vi "Trivial_client.vi"() -> (0 "Difference":dbl format="%.2f", 1 "Server time":dbl format="%.2f")   [LabVIEW 2020]
doc: "This is an example of using features of the VI Server as a client. It shows how you might browse from one or more applications that may be exporting data from one or more data stations. \n\nThe example shows how to query a server for its list of exported VIs, how to get references to the VIs, and how call them with the Call By Reference function."
uses:
  Anemometry/Anemometry Sub Vis/Globals/Preference_global.vi
panel:
  out "Iterations":i32
  out "error Out":errorcluster
  in  "trivial.vi type":refnum<vi>
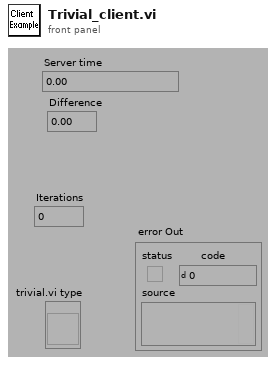
[diagram p1: front panel]
types:
  T1 = typedef "Server_Comms.ctl" = enum16{"Do Not Link To Server", "Server Link Healthy"}
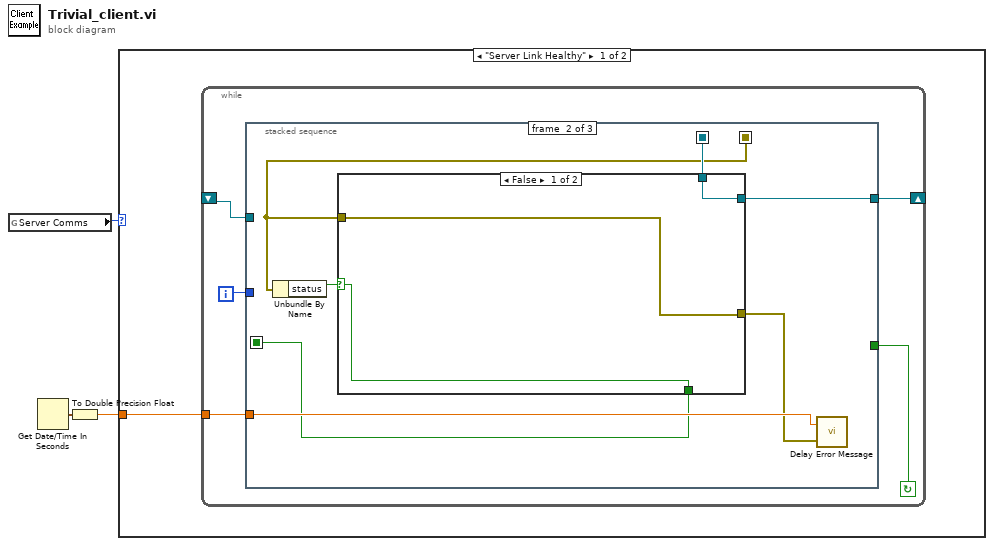
[diagram p0: block diagram]
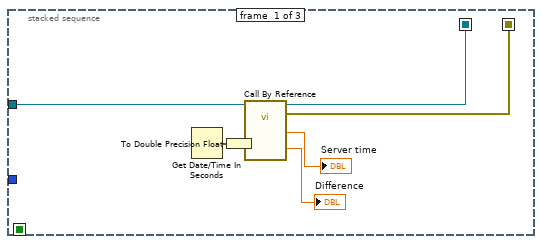
[diagram p2: hidden frame]
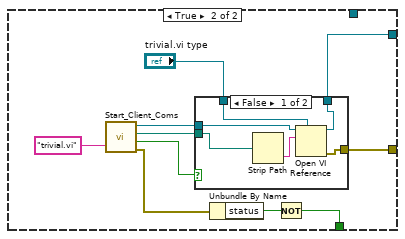
[diagram p3: hidden frame]
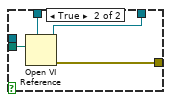
[diagram p4: hidden frame]
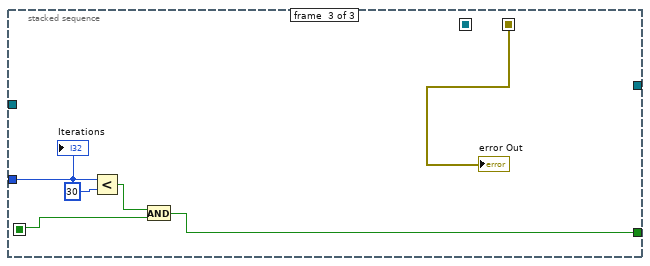
[diagram p5: hidden frame]
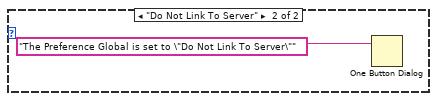
[diagram p6: hidden frame]
diagram:
  n1 = global read "Preference_global.vi" "Server Comms"() -> (w3:T1)
  n2 = Get Date/Time In Seconds() -> (seconds since 1Jan1904=w2:timestamp)
  n3 = To Double Precision Float(number=w2) -> (double precision float=w1:dbl)
  n4 = case shown="\"Server Link Healthy\"" w3 {
    tunnel: w1 -> [w4 _]
    frame "Server Link Healthy" {
      n5 = while {
        shift-left: _ -> [w9]
        shift-right: [w8] -> _
        tunnel: w4 -> [w5]
        i -> [w7]
        stop <- w6 continue-if-true
        n6 = stacked-sequence {
          seq-local: [w11 _ _] -> [_ w22 _]
          seq-local: [w13 _ _] -> [_ w20 w48]
          seq-local: [_ w17 _] -> [_ _ w49]
          tunnel: w9 -> [w12 _ _]
          tunnel: [_ w23 _] -> w8
          tunnel: w7 -> [_ _ w50]
          tunnel: [_ _ w47] -> w6
          tunnel: w5 -> [_ w19 _]
          frame #0 {
            n7 = Get Date/Time In Seconds() -> (seconds since 1Jan1904=w10:timestamp)
            n8 = To Double Precision Float(number=w10) -> (double precision float=w14:dbl)
            n9 = call-by-ref "?"(reference=w12, "Client time"=w14) -> (reference out=w11:refnum<vi>, error out=w13:errorcluster, "Server time"=→"Server time":dbl, "Difference"=→"Difference":dbl)  [unwired: 1 in]
          }
          frame #1 {
            n10 = Unbundle By Name(w20) -> ("status"=w21:bool)
            n11 = case shown="False" w21 {
              selector: w21 -> [w24 _]
              tunnel: [w26 w32] -> w23
              tunnel: w22 -> [w26 _]
              tunnel: [w25 w30] -> w18
              tunnel: w20 -> [w25 _]
              tunnel: [w24 w27] -> w17
              frame False {
              }
              frame True {
                n12 = call "Start_Client_Coms.vi"("VI name to run on server"="trivial.vi") -> ("LabVIEW application reference"=w34:refnum<vi>, "Checked VI name"=w31:path, "Local Call"=w33:bool, "Error cluster"=w28:errorcluster)  [unwired: 1 in]
                n13 = case shown="False" w33 {
                  tunnel: [w39 w46] -> w32
                  tunnel: "trivial.vi type" -> [w38 w45]
                  tunnel: w31 -> [w40 w44]
                  tunnel: w34 -> [w37 _]
                  tunnel: [w41 w43] -> w30
                  frame False {
                    n14 = Strip Path(path=w40) -> (name=w42:string)  [unwired: 1 out]
                    n15 = Open VI Reference(type specifier VI Refnum (for type only)=w38, application reference (local)=w37, vi path=w42) -> (vi reference=w39:refnum<vi>, error out=w41:errorcluster)  [unwired: 1 in, 2 out]
                  }
                  frame True {
                    n16 = Open VI Reference(type specifier VI Refnum (for type only)=w45, vi path=w44) -> (vi reference=w46:refnum<vi>, error out=w43:errorcluster)  [unwired: 1 in, 3 out]
                  }
                }
                n17 = Unbundle By Name(w28) -> ("status"=w29:bool)
                n18 = Not(x=w29) -> (.not. x?=w27:bool)
              }
            }
            n19 = call "Delay Error Message.vi"("error in (no error)"=w18, "Seconds since 1904"=w19) -> ()  [unwired: 2 in]
          }
          frame #2 {
            n20 = Less?(x=w50, y=30) -> (x < y?=w52:bool)
            n21 = And(x=w52, y=w49) -> (x .and. y?=w47:bool)
            "Iterations" <- w50
            "error Out" <- w48
          }
        }
      }
    }
    frame "Do Not Link To Server" {
      n22 = One Button Dialog(message="The Preference Global is set to \"Do Not Link To Server\"") -> ()  [unwired: 2 out]
    }
  }
